vi "testvmic.vi"() -> ()   [LabVIEW 2014]
uses:
  <instrlib>/niSync/niSync.llb/niSync Initialize (IVI).vi
  <userlib>/VMIC/VMIC 5565 Reflective Memory.llb/VMIC Write (U32).vi
  <userlib>/VMIC/VMIC 5565 Reflective Memory.llb/VMIC Read (U8).vi
panel:
  out "数组 2":sgl[](array[numeric])
  out "buffer 3":u32[](array[numeric])
  out "数组":dbl[](array[numeric])
  out "buffer 2":sgl[](array[numeric])
  out "error out 2":errorcluster
  out "error out":errorcluster {"code" format="%.0x"}
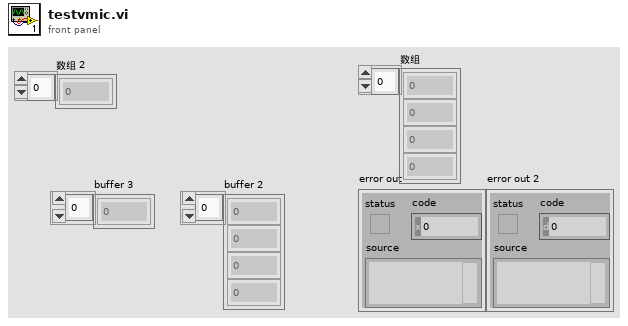
[diagram p1: front panel]
types:
  T1 = typedef "VMIC Reference.ctl" = variant
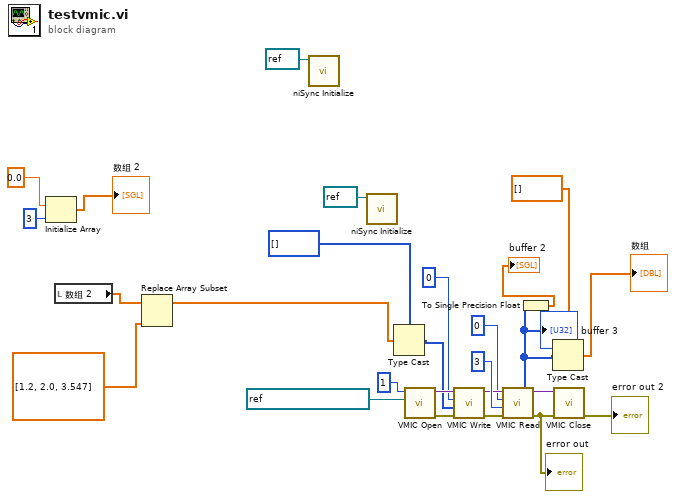
[diagram p0: block diagram]
diagram:
  n1 = Initialize Array(sgl 0.0, 3 ("维数大小")) -> (→"数组 2":sgl[])
  n2 = local read "数组 2"() -> (w3:sgl[])
  n3 = Replace Array Subset(array=w3, new element=dbl[] [1.2, 2.0, 3.547]) -> (w1:sgl[])  [unwired: 1 in]
  n4 = call-poly <instrlib>:"niSync Initialize.vi"("resource name"=refnum<k15> refnum) -> ()  [unwired: 9 in, 2 out]
  n5 = call-poly <instrlib>:"niSync Initialize.vi"("resource name"=refnum<k15> refnum) -> ()  [unwired: 9 in, 2 out]
  n6 = Type Cast(type=u32[] [], x=w1) -> (*(type *) &x=w12:u32[])
  n7 = call <userlib>:"VMIC Open.vi"("VISA resource name (empty)"=refnum<visa-resource-name> "PXI13::12::INSTR", "device (1)"=1) -> ("error out"=w23:errorcluster, "VMIC reference"=w24:T1)  [unwired: 4 in]
  n8 = call-poly <userlib>:"VMIC Write.vi"("error in (no error)"=w23, "buffer"=w12, "offset (0)"=u32 0, "VMIC reference in"=w24) -> ("error out"=w21:errorcluster, "VMIC reference out"=w19:T1)  [unwired: 2 in]
  n9 = call-poly <userlib>:"VMIC Read.vi"("error in (no error)"=w21, "length (0)"=u32 3, "offset (0)"=u32 0, "VMIC reference in"=w19) -> ("error out"=w17:errorcluster, "buffer"=w8:u32[], "VMIC reference out"=w18:T1)  [unwired: 1 in]
  "error out" <- w17
  "buffer 3" <- w8
  n10 = To Single Precision Float(number=w8) -> (single precision float=→"buffer 2":sgl[])
  n11 = Type Cast(type=sgl[] [], x=w8) -> (*(type *) &x=→"数组":sgl[])
  n12 = call <userlib>:"VMIC Close.vi"("error in (no error)"=w17, "VMIC reference in"=w18) -> ("error out"=→"error out 2":errorcluster)  [unwired: 5 in]
